vi "SetScanFormats.vi"(0 "Cluster":T2, 1 "Énum":T1, 3 "Répertoire initial":path=path "C:/Données/Run003", 5 "Scan Pref":string="Scan" caption="Prefixe Scan", 7 "UseSubFolder":bool, 9 "Log Pref":string="Log" caption="Prefixe Log", 11 "ErrorIn(No Error)":errorcluster caption="entrée d'erreur (pas d'erreur)", 12 "GraphConfig":i32, 14 "Experiment":path=path "C:/Données/Run003") -> (15 "sortie d'erreur":errorcluster)   [LabVIEW 2019]
uses:
  SetInitPar.ctl
  <vilib>/Utility/config.llb/Write Key (String).vi
  <vilib>/Utility/config.llb/Write Key (Boolean).vi
  <vilib>/Utility/config.llb/Write Key (I32).vi
  <vilib>/Utility/config.llb/Write Key (Path).vi
  <vilib>/Utility/config.llb/NI_LVConfig.lvlib
panel:
  in  "AllowSave":bool=TRUE
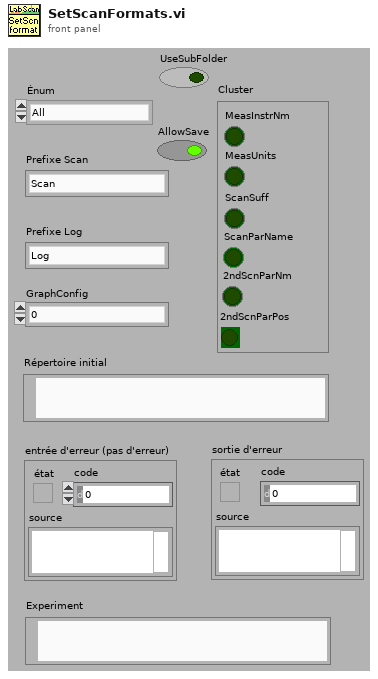
[diagram p1: front panel]
types:
  T1 = typedef "SetInitPar.ctl" = enum16{"All", "AllowSave", "GraphConfig", "ScanFormats", "ScanPref", "LogPref", "BasePath", "Experiment", "SubFolder"}
  T2 = cluster{"MeasInstrNm":bool, "MeasUnits":bool, "ScanSuff":bool, "ScanParNm":bool, "2ndScnParNm":bool, "2ndScnParPos":bool}
  T3 = typedef "NI_LVConfig.lvlib/Config Data RefNum.ctl" = refnum<k1>
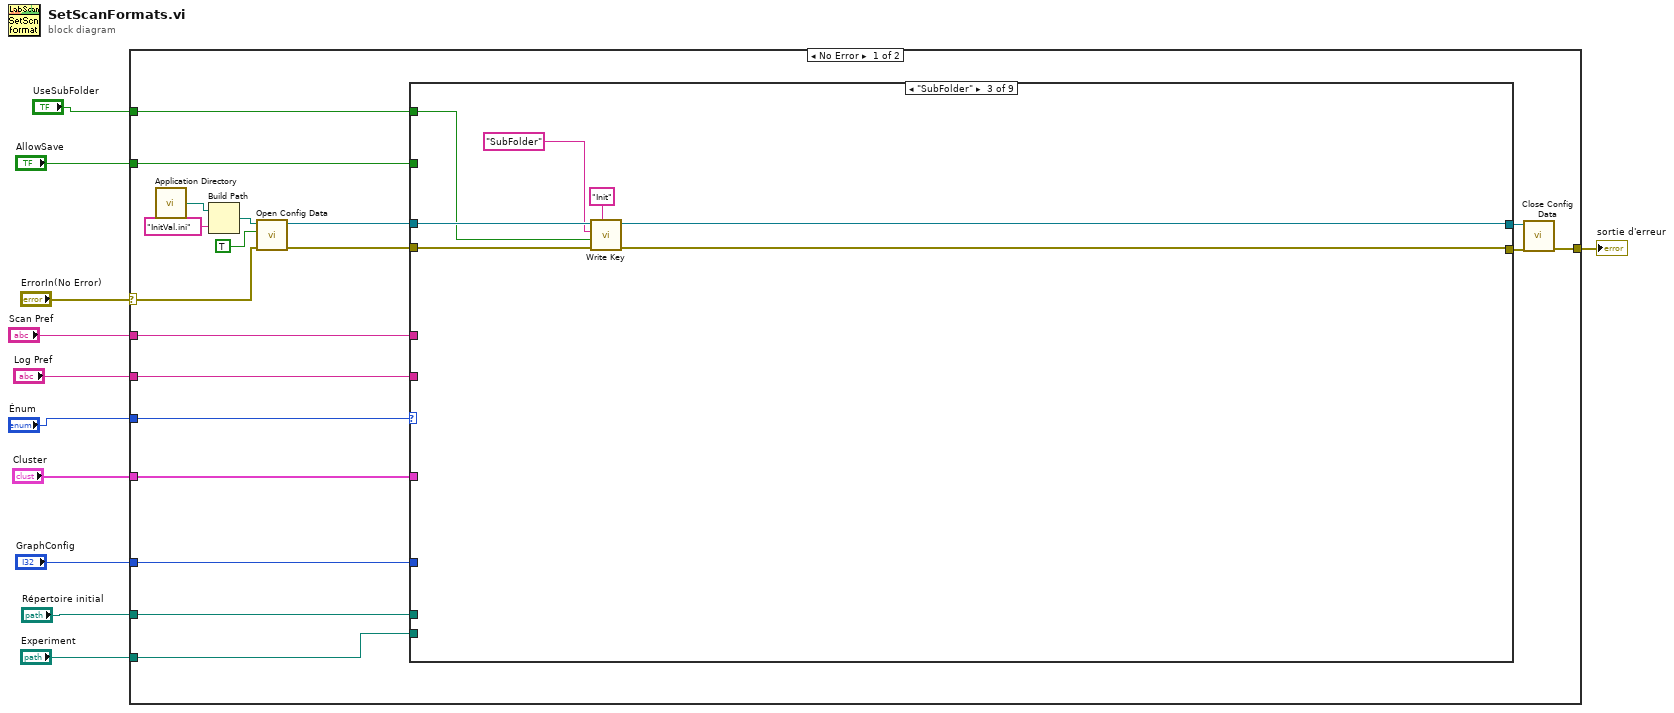
[diagram p0: block diagram]
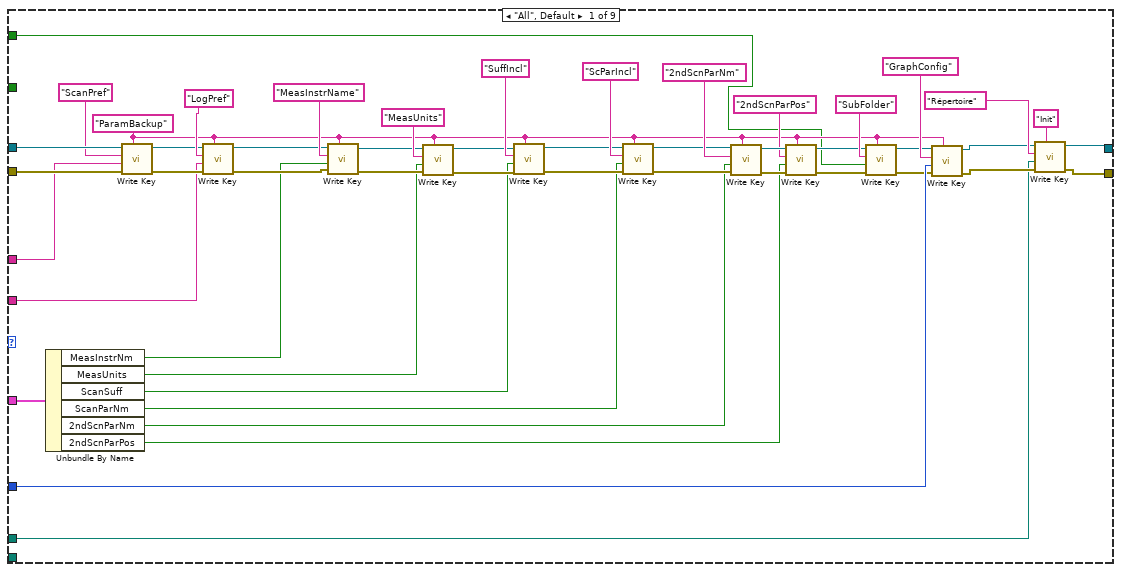
[diagram p2: hidden frame]
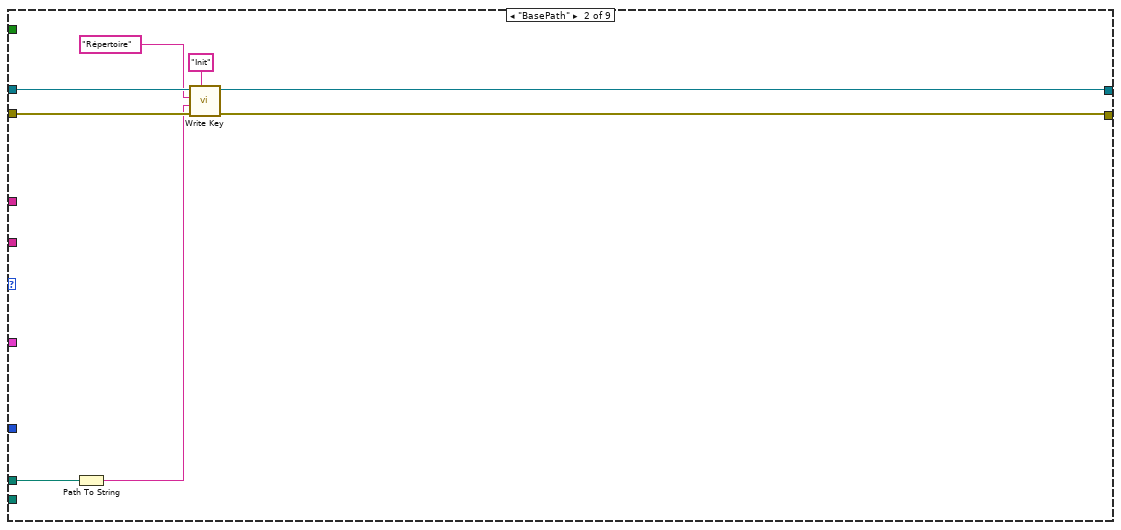
[diagram p3: hidden frame]
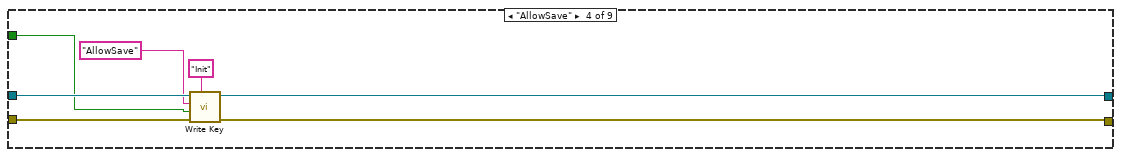
[diagram p4: hidden frame]
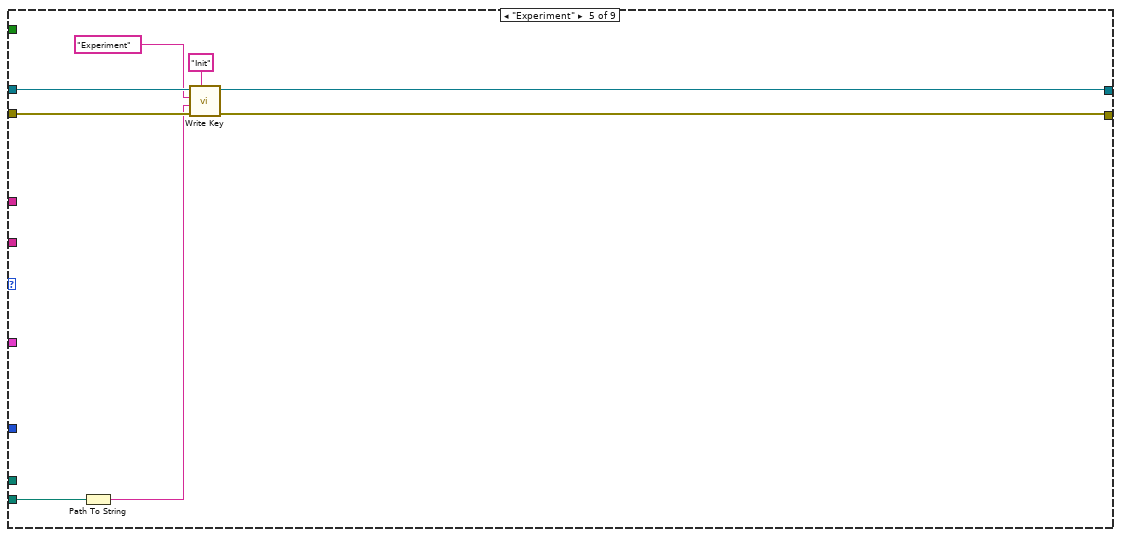
[diagram p5: hidden frame]
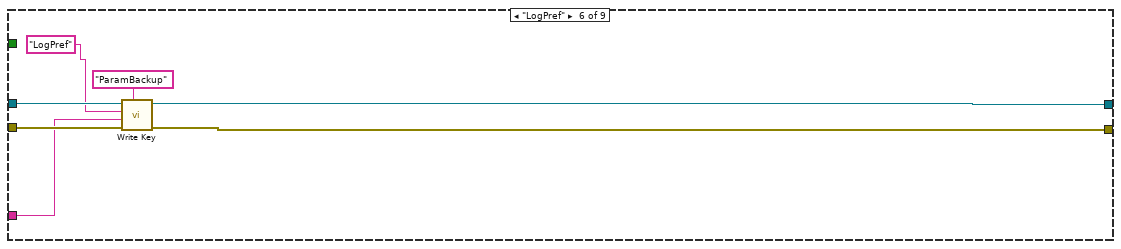
[diagram p6: hidden frame]
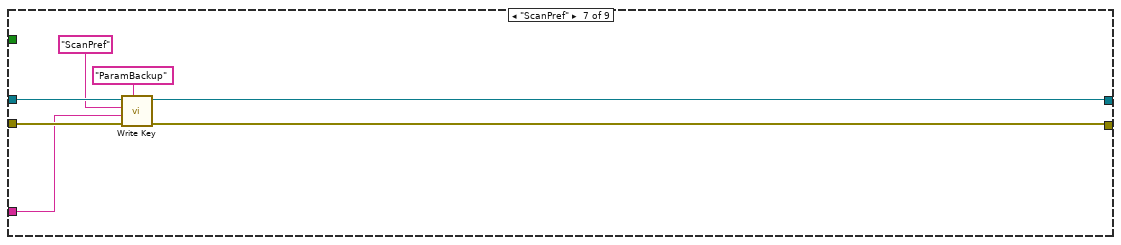
[diagram p7: hidden frame]
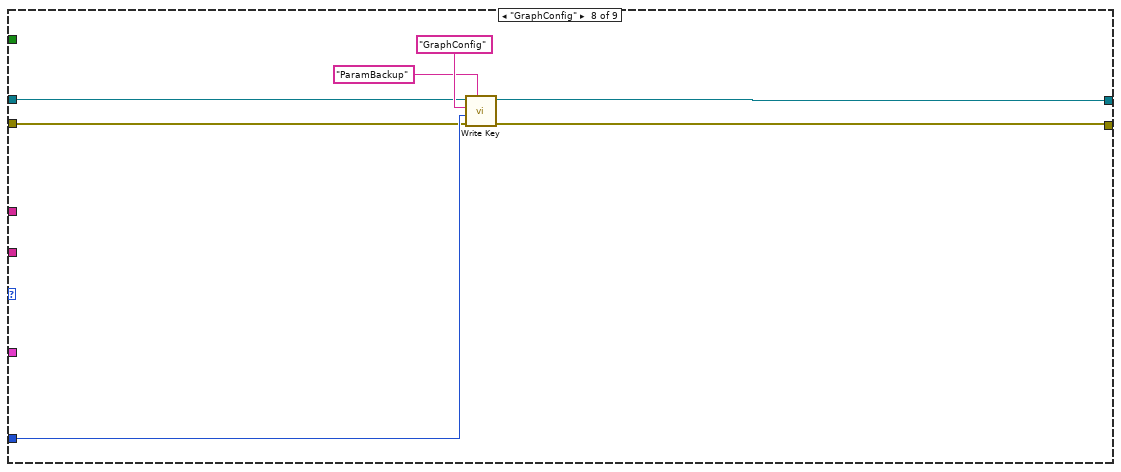
[diagram p8: hidden frame]
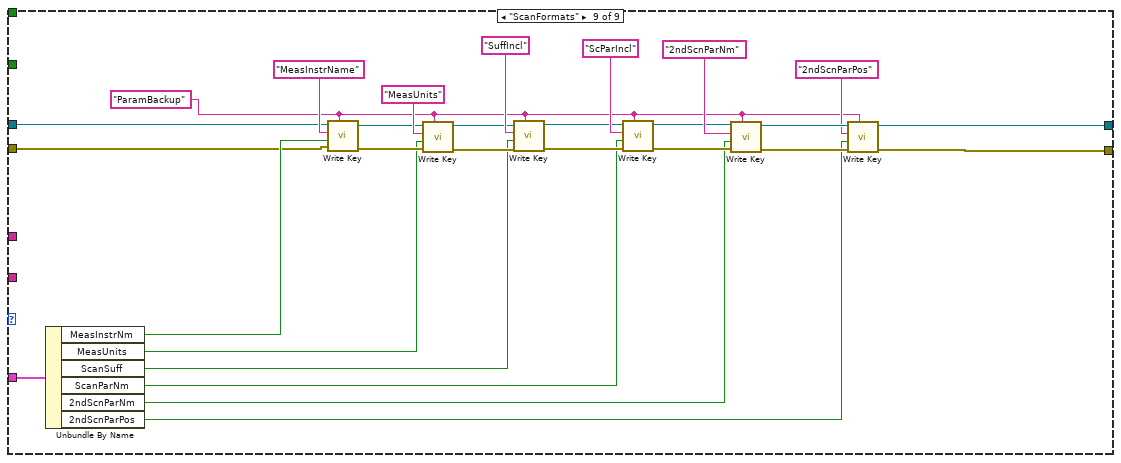
[diagram p9: hidden frame]
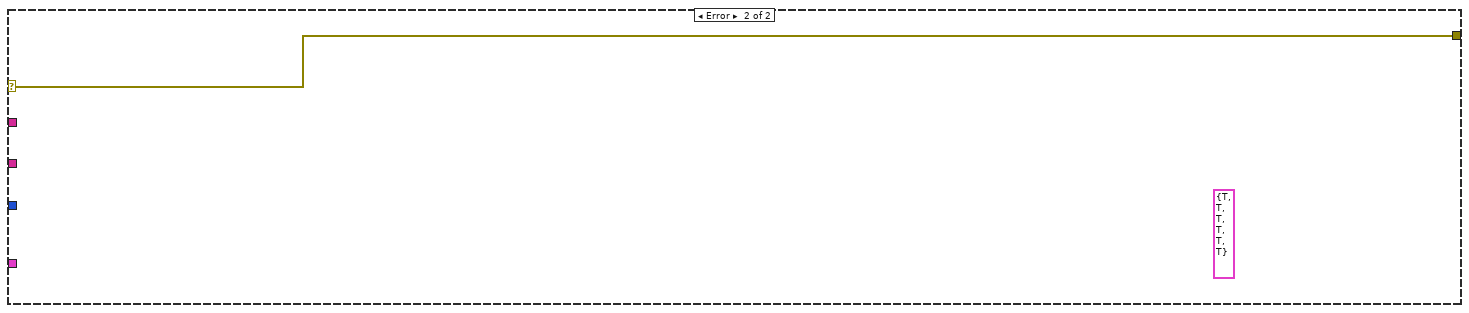
[diagram p10: hidden frame]
diagram:
  n1 = case shown="No Error" "ErrorIn(No Error)" {
    selector: "ErrorIn(No Error)" -> [w24 w159]
    tunnel: [w23 w159] -> w10
    tunnel: "Scan Pref" -> [w21 _]
    tunnel: "Cluster" -> [w22 _]
    tunnel: "Log Pref" -> [w20 _]
    tunnel: "GraphConfig" -> [w17 _]
    tunnel: "Énum" -> [w16 _]
    tunnel: "Répertoire initial" -> [w15 _]
    tunnel: "Experiment" -> [w14 _]
    tunnel: "AllowSave" -> [w13 _]
    tunnel: "UseSubFolder" -> [w12 _]
    frame No Error {
      n2 = call <vilib>:"Application Directory.vi"() -> ("Application Directory"=w28:path)
      n3 = Build Path(base path=w28, name or relative path="InitVal.ini") -> (appended path=w27:path)
      n4 = call <vilib>:"Open Config Data.vi"("error in (no error)"=w24, "create file if necessary (T)"=TRUE ("create file if necessary? (T)"), "configuration file path"=w27) -> ("error out"=w29:errorcluster, "refnum"=w30:T3)  [unwired: 6 in, 1 out]
      n5 = case shown="\"SubFolder\"" w16 {
        tunnel: w30 -> [w79 w87 w94 w101 w109 w116 w123 w126 w135]
        tunnel: w29 -> [w78 w86 w93 w100 w108 w115 w122 w125 w134]
        tunnel: w22 -> [w61 _ _ _ _ _ _ _ w142]
        tunnel: w21 -> [w60 _ _ _ _ w114 w121 _ _]
        tunnel: w20 -> [w55 _ _ _ _ _ _ _ _]
        tunnel: [w41 w81 w90 w96 w104 w111 w118 w130 w131] -> w19
        tunnel: [w39 w82 w91 w97 w105 w110 w117 w129 w132] -> w18
        tunnel: w17 -> [w45 _ _ _ _ _ _ w127 _]
        tunnel: w15 -> [w38 w83 _ _ _ _ _ _ _]
        tunnel: w14 -> [_ _ _ _ w103 _ _ _ _]
        tunnel: w13 -> [_ _ _ w95 _ _ _ _ _]
        tunnel: w12 -> [w31 _ w88 _ _ _ _ _ _]
        frame "All", Default {
          w35 = "ParamBackup"
          n6 = Unbundle By Name(w61) -> ("MeasInstrNm"=w54:bool, "MeasUnits"=w51:bool, "ScanSuff"=w50:bool, "ScanParNm"=w49:bool, "2ndScnParNm"=w48:bool, "2ndScnParPos"=w47:bool)
          n7 = call-poly <vilib>:"Write Key.vi"("section"=w35, "error in (no error)"=w78, "value"=w60, "key"="ScanPref", "refnum"=w79) -> ("error out"=w59:errorcluster, "refnum out"=w53:T3)  [unwired: 4 in, 1 out]
          n8 = call-poly <vilib>:"Write Key.vi"("section"=w35, "error in (no error)"=w59, "value"=w55, "key"="LogPref", "refnum"=w53) -> ("error out"=w58:errorcluster, "refnum out"=w52:T3)  [unwired: 4 in, 1 out]
          n9 = call-poly <vilib>:"Write Key.vi"("section"=w35, "error in (no error)"=w58, "value"=w54, "key"="MeasInstrName", "refnum"=w52) -> ("error out"=w68:errorcluster, "refnum out"=w66:T3)  [unwired: 4 in, 1 out]
          n10 = call-poly <vilib>:"Write Key.vi"("section"=w35, "error in (no error)"=w68, "value"=w51, "key"="MeasUnits", "refnum"=w66) -> ("error out"=w67:errorcluster, "refnum out"=w65:T3)  [unwired: 4 in, 1 out]
          n11 = call-poly <vilib>:"Write Key.vi"("section"=w35, "error in (no error)"=w67, "value"=w50, "key"="SuffIncl", "refnum"=w65) -> ("error out"=w71:errorcluster, "refnum out"=w72:T3)  [unwired: 4 in, 1 out]
          n12 = call-poly <vilib>:"Write Key.vi"("section"=w35, "error in (no error)"=w71, "value"=w49, "key"="ScParIncl", "refnum"=w72) -> ("error out"=w75:errorcluster, "refnum out"=w74:T3)  [unwired: 4 in, 1 out]
          n13 = call-poly <vilib>:"Write Key.vi"("section"=w35, "error in (no error)"=w75, "value"=w48, "key"="2ndScnParNm", "refnum"=w74) -> ("error out"=w64:errorcluster, "refnum out"=w63:T3)  [unwired: 4 in, 1 out]
          n14 = call-poly <vilib>:"Write Key.vi"("section"=w35, "error in (no error)"=w64, "value"=w47, "key"="2ndScnParPos", "refnum"=w63) -> ("error out"=w36:errorcluster, "refnum out"=w34:T3)  [unwired: 4 in, 1 out]
          n15 = call-poly <vilib>:"Write Key.vi"("section"=w35, "error in (no error)"=w36, "value"=w31, "key"="SubFolder", "refnum"=w34) -> ("error out"=w32:errorcluster, "refnum out"=w33:T3)  [unwired: 4 in, 1 out]
          n16 = call-poly <vilib>:"Write Key.vi"("section"=w35, "error in (no error)"=w32, "value"=w45, "key"="GraphConfig", "refnum"=w33) -> ("error out"=w42:errorcluster, "refnum out"=w40:T3)  [unwired: 4 in, 1 out]
          n17 = call-poly <vilib>:"Write Key.vi"("section"="Init", "error in (no error)"=w42, "value"=w38, "key"="Répertoire", "refnum"=w40) -> ("error out"=w41:errorcluster, "refnum out"=w39:T3)  [unwired: 4 in, 1 out]
        }
        frame "BasePath" {
          n18 = Path To String(path=w83) -> (string=w80:string)
          n19 = call-poly <vilib>:"Write Key.vi"("section"="Init", "error in (no error)"=w86, "value"=w80, "key"="Répertoire", "refnum"=w87) -> ("error out"=w81:errorcluster, "refnum out"=w82:T3)  [unwired: 4 in, 1 out]
        }
        frame "SubFolder" {
          n20 = call-poly <vilib>:"Write Key.vi"("section"="Init", "error in (no error)"=w93, "value"=w88, "key"="SubFolder", "refnum"=w94) -> ("error out"=w90:errorcluster, "refnum out"=w91:T3)  [unwired: 4 in, 1 out]
        }
        frame "AllowSave" {
          n21 = call-poly <vilib>:"Write Key.vi"("section"="Init", "error in (no error)"=w100, "value"=w95, "key"="AllowSave", "refnum"=w101) -> ("error out"=w96:errorcluster, "refnum out"=w97:T3)  [unwired: 4 in, 1 out]
        }
        frame "Experiment" {
          n22 = Path To String(path=w103) -> (string=w102:string)
          n23 = call-poly <vilib>:"Write Key.vi"("section"="Init", "error in (no error)"=w108, "value"=w102, "key"="Experiment", "refnum"=w109) -> ("error out"=w104:errorcluster, "refnum out"=w105:T3)  [unwired: 4 in, 1 out]
        }
        frame "LogPref" {
          n24 = call-poly <vilib>:"Write Key.vi"("section"="ParamBackup", "error in (no error)"=w115, "value"=w114, "key"="LogPref", "refnum"=w116) -> ("error out"=w111:errorcluster, "refnum out"=w110:T3)  [unwired: 4 in, 1 out]
        }
        frame "ScanPref" {
          n25 = call-poly <vilib>:"Write Key.vi"("section"="ParamBackup", "error in (no error)"=w122, "value"=w121, "key"="ScanPref", "refnum"=w123) -> ("error out"=w118:errorcluster, "refnum out"=w117:T3)  [unwired: 4 in, 1 out]
        }
        frame "GraphConfig" {
          n26 = call-poly <vilib>:"Write Key.vi"("section"="ParamBackup", "error in (no error)"=w125, "value"=w127, "key"="GraphConfig", "refnum"=w126) -> ("error out"=w130:errorcluster, "refnum out"=w129:T3)  [unwired: 4 in, 1 out]
        }
        frame "ScanFormats" {
          w133 = "ParamBackup"
          n27 = Unbundle By Name(w142) -> ("MeasInstrNm"=w141:bool, "MeasUnits"=w140:bool, "ScanSuff"=w139:bool, "ScanParNm"=w138:bool, "2ndScnParNm"=w137:bool, "2ndScnParPos"=w136:bool)
          n28 = call-poly <vilib>:"Write Key.vi"("section"=w133, "error in (no error)"=w134, "value"=w141, "key"="MeasInstrName", "refnum"=w135) -> ("error out"=w149:errorcluster, "refnum out"=w147:T3)  [unwired: 4 in, 1 out]
          n29 = call-poly <vilib>:"Write Key.vi"("section"=w133, "error in (no error)"=w149, "value"=w140, "key"="MeasUnits", "refnum"=w147) -> ("error out"=w148:errorcluster, "refnum out"=w146:T3)  [unwired: 4 in, 1 out]
          n30 = call-poly <vilib>:"Write Key.vi"("section"=w133, "error in (no error)"=w148, "value"=w139, "key"="SuffIncl", "refnum"=w146) -> ("error out"=w152:errorcluster, "refnum out"=w153:T3)  [unwired: 4 in, 1 out]
          n31 = call-poly <vilib>:"Write Key.vi"("section"=w133, "error in (no error)"=w152, "value"=w138, "key"="ScParIncl", "refnum"=w153) -> ("error out"=w156:errorcluster, "refnum out"=w155:T3)  [unwired: 4 in, 1 out]
          n32 = call-poly <vilib>:"Write Key.vi"("section"=w133, "error in (no error)"=w156, "value"=w137, "key"="2ndScnParNm", "refnum"=w155) -> ("error out"=w145:errorcluster, "refnum out"=w144:T3)  [unwired: 4 in, 1 out]
          n33 = call-poly <vilib>:"Write Key.vi"("section"=w133, "error in (no error)"=w145, "value"=w136, "key"="2ndScnParPos", "refnum"=w144) -> ("error out"=w131:errorcluster, "refnum out"=w132:T3)  [unwired: 4 in, 1 out]
        }
      }
      n34 = call <vilib>:"Close Config Data.vi"("error in (no error)"=w19, "refnum"=w18) -> ("error out"=w23:errorcluster)  [unwired: 8 in, 1 out]
    }
    frame Error {
      (unwired) T2 {"MeasInstrNm"=TRUE, "MeasUnits"=TRUE, "ScanSuff"=TRUE, "ScanParNm"=TRUE, "2ndScnParNm"=TRUE, "2ndScnParPos"=TRUE} ("Cluster")
    }
  }
  "sortie d'erreur" <- w10
